vi "Dispense.vi"(6 "Count":i32, 8 "error in (no error)":errorcluster, 11 "SoldState in":refnum<class "SoldState.lvclass">) -> (0 "error out":errorcluster, 1 "NextState":T1=enum."有硬幣", 2 "ProcessMessage":string, 3 "SoldState out":refnum<class "SoldState.lvclass">, 4 "Count Out":i32)   [LabVIEW 2013, in "SoldState.lvclass"]
uses:
  SoldState.lvclass
  StateMark.ctl
panel:
  # "糖果發放動作"
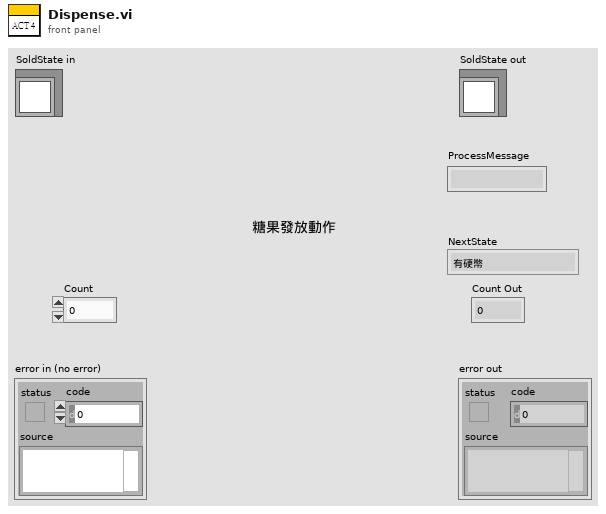
[diagram p1: front panel]
types:
  T1 = typedef "StateMark.ctl" = enum16{"沒有硬幣", "有硬幣", "賣出糖果", "糖果賣完", "NoChange"}
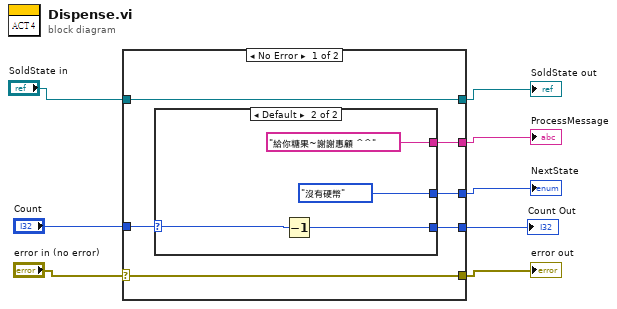
[diagram p0: block diagram]
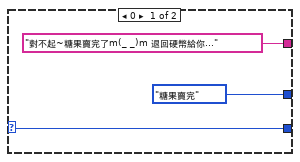
[diagram p2: hidden frame]
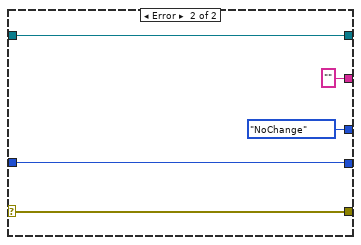
[diagram p3: hidden frame]
diagram:
  n1 = case shown="No Error" "error in (no error)" {
    selector: "error in (no error)" -> [w13 w25]
    tunnel: [w14 w26] -> w6
    tunnel: "SoldState in" -> [w14 w26]
    tunnel: [w13 w25] -> w1
    tunnel: [w12 "" ("ProcessMessage")] -> w5
    tunnel: [w11 StateMark."NoChange" ("NextState")] -> w3
    tunnel: "Count" -> [w10 w22]
    tunnel: [w9 w22] -> w2
    frame No Error {
      n2 = case shown="Default" w10 {
        selector: w10 -> [w15 w19]
        tunnel: ["對不起~糖果賣完了m(_ _)m 退回硬幣給你..." ("ProcessMessage") "給你糖果~謝謝惠顧 ^^" ("ProcessMessage")] -> w12
        tunnel: [StateMark."糖果賣完" ("NextState") StateMark."沒有硬幣" ("NextState")] -> w11
        tunnel: [w15 w18] -> w9
        frame 0 {
        }
        frame Default {
          n3 = Decrement(x=w19) -> (x-1=w18:i32)
        }
      }
    }
    frame Error {
    }
  }
  "error out" <- w1
  "SoldState out" <- w6
  "NextState" <- w3
  "ProcessMessage" <- w5
  "Count Out" <- w2
